vi "Get Terminal Refs for New Frame.vi"(8 "error in (no error)":errorcluster, 10 "Case Structure Ref":refnum<vi>, 11 "Getter Generator":refnum<class "Getter Generator.lvclass">) -> (0 "error out":errorcluster, 2 "reference out":refnum<vi>, 3 "Getter Generator 2":refnum<class "Getter Generator.lvclass">)   [LabVIEW 2020, in "Method Generation.lvlib" / "Getter Generator.lvclass"]
uses:
  Getter Generator.lvclass
  Getter Generator.lvclass/Getter Generator.ctl
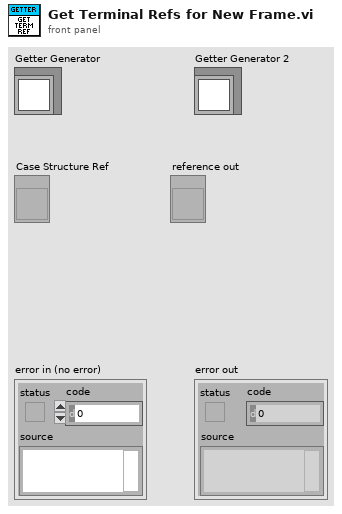
[diagram p1: front panel]
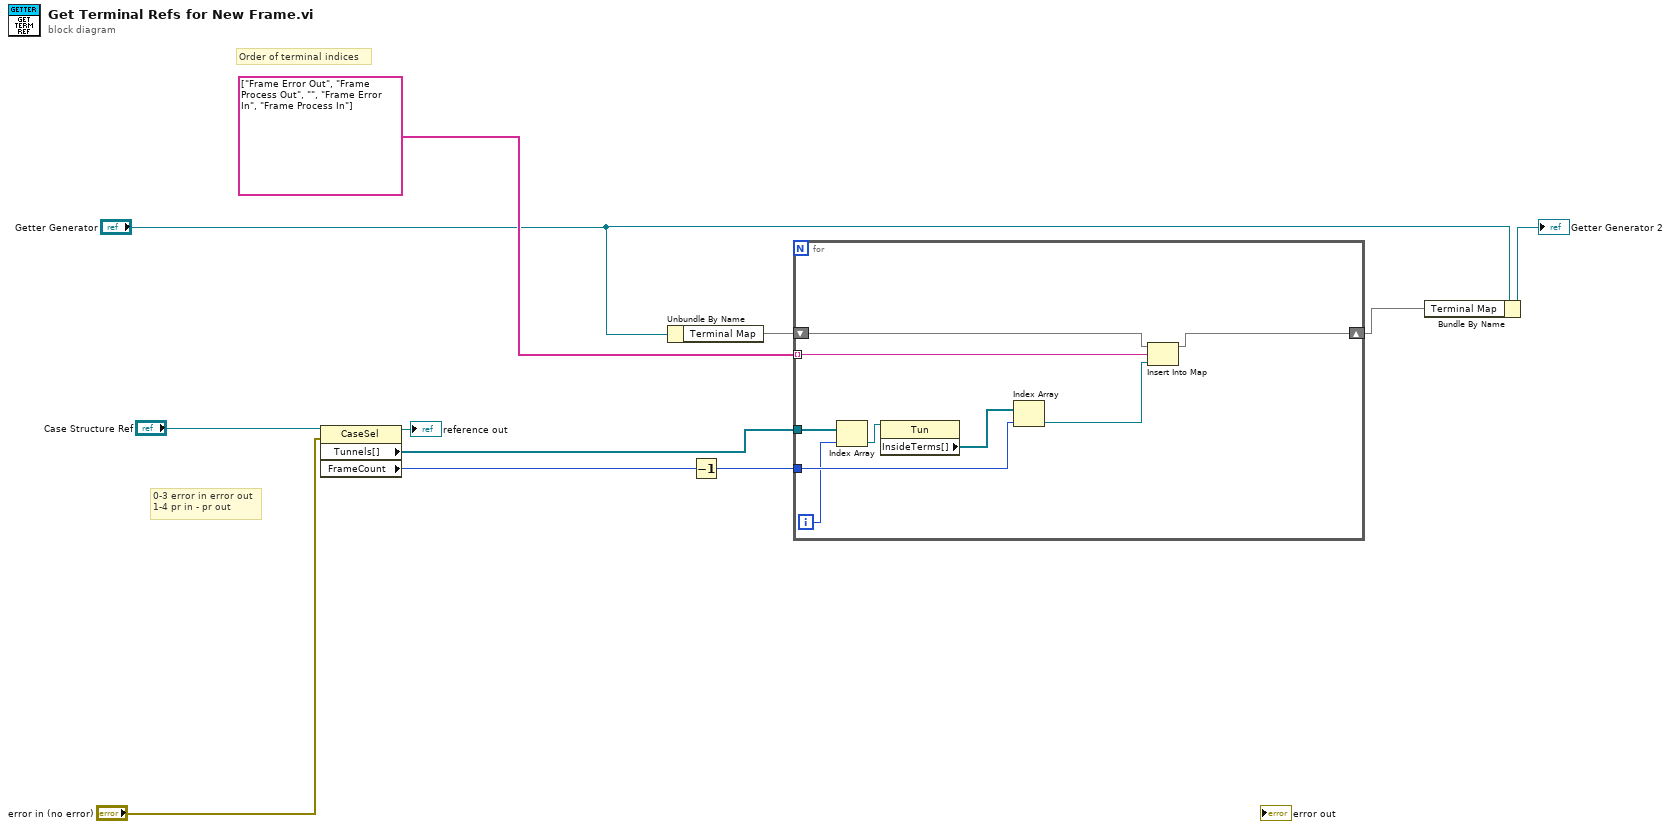
[diagram p0: block diagram]
diagram:
  # "Order of terminal indices"
  # "0-3 error in error out\n1-4 pr in - pr out"
  n1 = property class="CaseSel"(reference="Case Structure Ref", error in="error in (no error)") -> (reference out=→"reference out":refnum<vi>, "Tunnels[]"=w9:refnum<vi>[], "FrameCount"=w2:i32)  [unwired: 1 out]
  n2 = Unbundle By Name("Getter Generator") -> ("Terminal Map"=w4:map{string, refnum<vi>})
  n3 = Decrement(x=w2) -> (x-1=w8:i32)
  n4 = for {
    tunnel: w9 -> [w19]
    tunnel: w8 -> [w17]
    tunnel: string[] ["Frame Error Out", "Frame Process Out", "", "Frame Error In", "Frame Process In"] -> [w14] mode=indexing
    shift-right: [w12] -> w3
    shift-left: w4 -> [w15]
    i -> [w16]
    n5 = Index Array(array=w19, index=w16) -> (element=w20:refnum<vi>)
    n6 = property class="Tun"(reference=w20) -> ("InsideTerms[]"=w18:refnum<vi>[])  [unwired: 1 in, 2 out]
    n7 = Index Array(array=w18, index=w17) -> (element=w13:refnum<vi>)
    n8 = Insert Into Map(map in=w15, key=w14, value=w13) -> (map out=w12:map{string, refnum<vi>})  [unwired: 2 out]
  }
  n9 = Bundle By Name(cluster="Getter Generator", "Terminal Map"=w3) -> (→"Getter Generator 2":refnum<class "Getter Generator.lvclass">)
